vi "Sequencer Main - Copy.vi"() -> ()   [LabVIEW 2018] (continued)
                                # "Step TEST Result"
                                }
                                }
                                n2596 = global read "Global Variable.vi" "Array Errors"() -> (w5395:errorcluster[])
                                n2597 = Replace Array Subset(array=w5395, new element=w5392, index=3) -> (w5394:errorcluster[])
                                n2598 = global write "Global Variable.vi" "Array Errors"(w5394) -> ()
                                }
                              }
                            }
                            frame "capmem_get" {
                              # "Parameters"
                              # "Cmd"
                              n2599 = To Word Integer(number=w5406) -> (16bit integer=w5405:i16)
                              n2600 = To Word Integer(number=w5407) -> (16bit integer=w5404:i16)
                              n2601 = flat-sequence {
                                tunnel: [w5416] -> w5410
                                tunnel: [w5414] -> w5409
                                tunnel: [w5415] -> w5408
                                tunnel: w5410 -> [w5429]
                                tunnel: w5409 -> [w5428]
                                tunnel: w5408 -> [w5423]
                                tunnel: w5404 -> [w5427]
                                tunnel: w5405 -> [w5426]
                                tunnel: [w5425] -> w5403
                                tunnel: [w5424] -> w5402
                                tunnel: [w5422] -> w5399
                                tunnel: [w5421] -> w5398
                                frame #0 {
                                n2602 = global read "Global Variable.vi" "COM Port FTDI RS232"() -> (w5417:refnum<visa-resource-name>)
                                n2603 = call "ADB-Serial_WrRd.vi"("Timeout(Sec)"=1.0, "PassString"="Chuck(3)", "Command"="capmem", "ComPort"=w5417) -> ("error out"=w5415:errorcluster, "PASS"=w5416:bool, "received"=w5414:string)  [unwired: 5 in]
                                }
                                frame #1 {
                                n2604 = case shown="False" w5429 {
                                tunnel: w5428 -> [w5430 w5434]
                                tunnel: w5427 -> [_ w5439]
                                tunnel: w5426 -> [_ w5438]
                                tunnel: [FALSE w5437] -> w5425
                                tunnel: [w5432 w5436] -> w5424
                                tunnel: w5423 -> [w5432 w5436]
                                tunnel: [-1 w5435] -> w5422
                                tunnel: [w5430 w5434] -> w5421
                                frame False {
                                }
                                frame True {
                                n2605 = invoke on="Serial CMD Mon" class="Str" method="Append String"("string"=w5434) -> ()  [unwired: 3 in, 4 out]
                                n2606 = Match Pattern(string=w5434, regular expression="voltage") -> (after substring=w5443:string)  [unwired: 1 in, 3 out]
                                n2607 = Scan From String(format string="%d", input string=w5443, initial scan location=u32 0) -> (output 1=w5435:i32)  [unwired: 2 in, 3 out]
                                n2608 = In Range and Coerce(upper limit=w5439, x=w5435, lower limit=w5438) -> (In Range?=w5437:bool)  [unwired: 1 out]
                                }
                                }
                                }
                              }
                              n2609 = global read "Global Variable.vi" "Array Errors"() -> (w5411:errorcluster[])
                              n2610 = Replace Array Subset(array=w5411, new element=w5402, index=3) -> (w5412:errorcluster[])
                              n2611 = global write "Global Variable.vi" "Array Errors"(w5412) -> ()
                              n2612 = case shown="True" w5403 {
                                tunnel: [enum16{"Idle", "PASS", "FALSE"}."FALSE" ("Step Test Result") enum16{"Idle", "PASS", "FALSE"}."PASS" ("Step Test Result")] -> w5401
                                frame False {
                                # "Step TEST Result"
                                }
                                frame True {
                                # "Step TEST Result"
                                }
                              }
                              n2613 = Number To Decimal String(number=w5399) -> (decimal integer string=w5400:string)  [unwired: 1 in]
                            }
                            frame "setPowerRes" {
                              # "Param"
                              # "Cmd"
                              n2614 = flat-sequence {
                                tunnel: [w5457] -> w5452
                                tunnel: [w5456] -> w5451
                                tunnel: [w5455] -> w5450
                                tunnel: w5449 -> [w5454]
                                tunnel: w5452 -> [w5474]
                                tunnel: w5451 -> [w5475]
                                tunnel: [w5471] -> w5448
                                tunnel: w5450 -> [w5469]
                                tunnel: [w5470] -> w5447
                                tunnel: [w5469] -> w5446
                                frame #0 {
                                n2615 = for {
                                N: 1 -> [_]
                                tunnel: [w5459] -> w5457
                                tunnel: [w5468] -> w5456
                                shift-right: [w5458] -> w5455
                                shift-left: w5454 -> [w5463]
                                stop <- w5459 stop-if-true
                                n2616 = call <vilib>:"Space Constant.vi"() -> ("String"=w5462:string)
                                n2617 = global read "Global Variable.vi" "COM Port FTDI RS232"() -> (w5467:refnum<visa-resource-name>)
                                n2618 = Concatenate Strings("setPowerRes", w5462, w5463) -> (w5461:string)
                                n2619 = call "ADB-Serial_WrRd.vi"("Timeout(Sec)"=2.0, "PassString"="Set power resistor", "Command"=w5461, "ComPort"=w5467) -> ("error out"=w5468:errorcluster, "PASS"=w5459:bool, "received"=w5458:string)  [unwired: 5 in]
                                n2620 = invoke on="Serial CMD Mon" class="Str" method="Append String"("string"=w5458) -> ()  [unwired: 3 in, 4 out]
                                n2621 = Wait (ms)(milliseconds to wait=u32 500) -> ()  [unwired: 1 out]
                                }
                                }
                                frame #1 {
                                n2622 = global read "Global Variable.vi" "Array Errors"() -> (w5478:errorcluster[])
                                n2623 = call <userlib>:"Multi-line String to Array__ogtk.vi"("string"=w5469) -> ("lines"=w5473:string[])
                                n2624 = case shown="False" w5474 {
                                tunnel: [enum16{"Idle", "PASS", "FALSE"}."FALSE" ("Step Test Result") enum16{"Idle", "PASS", "FALSE"}."PASS" ("Step Test Result")] -> w5471
                                frame False {
                                # "Step TEST Result"
                                }
                                frame True {
                                # "Step TEST Result"
                                }
                                }
                                n2625 = Replace Array Subset(array=w5478, new element=w5475, index=3) -> (w5477:errorcluster[])
                                n2626 = Index Array(array=w5473, index=2 ("line index")) -> (element=w5470:string)
                                n2627 = global write "Global Variable.vi" "Array Errors"(w5477) -> ()
                                }
                              }
                            }
                            frame "calibADCoffset" {
                              # "Param"
                              # "Cmd"
                              n2628 = flat-sequence {
                                tunnel: [w5489] -> w5485
                                tunnel: [w5488] -> w5484
                                tunnel: [w5486] -> w5483
                                tunnel: w5485 -> [w5501]
                                tunnel: w5484 -> [w5502]
                                tunnel: [w5503] -> w5482
                                tunnel: w5483 -> [w5499]
                                tunnel: [w5499] -> w5481
                                frame #0 {
                                n2629 = for {
                                N: 1 -> [_]
                                tunnel: [w5493] -> w5489
                                tunnel: [w5498] -> w5488
                                tunnel: [w5490] -> w5486
                                stop <- w5493 stop-if-true
                                n2630 = global read "Global Variable.vi" "COM Port FTDI RS232"() -> (w5497:refnum<visa-resource-name>)
                                n2631 = global write "Global Variable.vi" "ADC Offset"(0 ("ADC Offset")) -> ()
                                n2632 = call "ADB-Serial_WrRd.vi"("Timeout(Sec)"=2.0, "PassString"="Chuck(3)", "Command"="calibADCoffset", "ComPort"=w5497) -> ("error out"=w5498:errorcluster, "PASS"=w5493:bool, "received"=w5490:string)  [unwired: 5 in]
                                n2633 = invoke on="Serial CMD Mon" class="Str" method="Append String"("string"=w5490) -> ()  [unwired: 3 in, 4 out]
                                n2634 = Wait (ms)(milliseconds to wait=u32 200) -> ()  [unwired: 1 out]
                                }
                                }
                                frame #1 {
                                n2635 = case shown="True" w5501 {
                                tunnel: w5499 -> [_ w5513]
                                tunnel: [FALSE w5508] -> w5500
                                frame False {
                                }
                                frame True {
                                n2636 = Match Pattern(string=w5513, regular expression="New ADC offset:") -> (after substring=w5511:string)  [unwired: 1 in, 3 out]
                                n2637 = Scan From String(format string="%d", input string=w5511) -> (output 1=w5509:i32)  [unwired: 3 in, 3 out]
                                n2638 = global write "Global Variable.vi" "ADC Offset"(w5509) -> ()
                                n2639 = Greater Than 0?(x=w5509) -> (x > 0?=w5508:bool)
                                }
                                }
                                n2640 = global read "Global Variable.vi" "Array Errors"() -> (w5506:errorcluster[])
                                n2641 = Replace Array Subset(array=w5506, new element=w5502, index=3) -> (w5505:errorcluster[])
                                n2642 = case shown="False" w5500 {
                                tunnel: [enum16{"Idle", "PASS", "FALSE"}."FALSE" ("Step Test Result") enum16{"Idle", "PASS", "FALSE"}."PASS" ("Step Test Result")] -> w5503
                                frame False {
                                # "Step TEST Result"
                                }
                                frame True {
                                # "Step TEST Result"
                                }
                                }
                                n2643 = global write "Global Variable.vi" "Array Errors"(w5505) -> ()
                                }
                              }
                            }
                            frame "calibCCRsave" {
                              # "Param"
                              # "Cmd"
                              n2644 = flat-sequence {
                                tunnel: [w5525] -> w5520
                                tunnel: [w5524] -> w5519
                                tunnel: w5518 -> [w5522]
                                tunnel: [w5521] -> w5516
                                tunnel: w5520 -> [w5539]
                                tunnel: w5519 -> [w5540]
                                tunnel: [w5537] -> w5517
                                frame #0 {
                                n2645 = for {
                                N: 1 -> [_]
                                tunnel: [w5531] -> w5525
                                tunnel: [w5536] -> w5524
                                tunnel: w5522 -> [w5528]
                                tunnel: [w5527] -> w5521
                                stop <- w5531 stop-if-true
                                (unwired) ""
                                n2646 = global read "Global Variable.vi" "COM Port FTDI RS232"() -> (w5535:refnum<visa-resource-name>)
                                n2647 = call <vilib>:"Space Constant.vi"() -> ("String"=w5526:string)
                                n2648 = Concatenate Strings("calibCCRsave", w5526, w5528) -> (w5529:string)
                                n2649 = call "ADB-Serial_WrRd.vi"("Timeout(Sec)"=2.0, "PassString"="Chuck(3)", "Command"=w5529, "ComPort"=w5535) -> ("error out"=w5536:errorcluster, "PASS"=w5531:bool, "received"=w5527:string)  [unwired: 5 in]
                                n2650 = invoke on="Serial CMD Mon" class="Str" method="Append String"("string"=w5527) -> ()  [unwired: 3 in, 4 out]
                                n2651 = Wait (ms)(milliseconds to wait=u32 200) -> ()  [unwired: 1 out]
                                }
                                }
                                frame #1 {
                                n2652 = global read "Global Variable.vi" "Array Errors"() -> (w5543:errorcluster[])
                                n2653 = case shown="True" w5539 {
                                tunnel: [FALSE w5545] -> w5538
                                frame False {
                                }
                                frame True {
                                n2654 = global read "Global Variable.vi" "ADC Offset"() -> (w5546:i32)
                                n2655 = Greater Than 0?(x=w5546) -> (x > 0?=w5545:bool)
                                }
                                }
                                n2656 = Replace Array Subset(array=w5543, new element=w5540, index=3) -> (w5542:errorcluster[])
                                n2657 = global write "Global Variable.vi" "Array Errors"(w5542) -> ()
                                n2658 = case shown="False" w5538 {
                                tunnel: [enum16{"Idle", "PASS", "FALSE"}."FALSE" ("Step Test Result") enum16{"Idle", "PASS", "FALSE"}."PASS" ("Step Test Result")] -> w5537
                                frame False {
                                # "Step TEST Result"
                                }
                                frame True {
                                # "Step TEST Result"
                                }
                                }
                                }
                              }
                            }
                            frame "start_ble" {
                              # "Param"
                              # "Cmd"
                              n2659 = flat-sequence {
                                tunnel: [w5558] -> w5554
                                tunnel: [w5557] -> w5553
                                tunnel: [w5555] -> w5551
                                tunnel: [w5555] -> w5549
                                tunnel: w5554 -> [w5571]
                                tunnel: w5553 -> [w5572]
                                tunnel: [w5573] -> w5552
                                tunnel: w5551 -> [w5570]
                                tunnel: [w5568] -> w5550
                                frame #0 {
                                n2660 = for {
                                N: 1 -> [_]
                                tunnel: [w5561] -> w5558
                                tunnel: [w5566] -> w5557
                                tunnel: [w5559] -> w5555
                                stop <- w5561 stop-if-true
                                n2661 = global read "Global Variable.vi" "COM Port FTDI RS232"() -> (w5565:refnum<visa-resource-name>)
                                n2662 = call "ADB-Serial_WrRd.vi"("Timeout(Sec)"=7.0, "PassString"="Chuck(3)", "Command"="start_ble", "ComPort"=w5565) -> ("error out"=w5566:errorcluster, "PASS"=w5561:bool, "received"=w5559:string)  [unwired: 5 in]
                                n2663 = invoke on="Serial CMD Mon" class="Str" method="Append String"("string"=w5559) -> ()  [unwired: 3 in, 4 out]
                                n2664 = Wait (ms)(milliseconds to wait=u32 200) -> ()  [unwired: 1 out]
                                }
                                }
                                frame #1 {
                                n2665 = global read "Global Variable.vi" "Array Errors"() -> (w5576:errorcluster[])
                                n2666 = call <userlib>:"Multi-line String to Array__ogtk.vi"("string"=w5570) -> ("lines"=w5569:string[])
                                n2667 = Index Array(array=w5569, index=4) -> (element=w5568:string)
                                n2668 = Replace Array Subset(array=w5576, new element=w5572, index=3) -> (w5575:errorcluster[])
                                n2669 = global write "Global Variable.vi" "Array Errors"(w5575) -> ()
                                n2670 = case shown="False" w5571 {
                                tunnel: [enum16{"Idle", "PASS", "FALSE"}."FALSE" ("Step Test Result") enum16{"Idle", "PASS", "FALSE"}."PASS" ("Step Test Result")] -> w5573
                                frame False {
                                # "Step TEST Result"
                                }
                                frame True {
                                # "Step TEST Result"
                                }
                                }
                                }
                              }
                            }
                            frame "setopvg" {
                              # "Param"
                              # "Cmd"
                              n2671 = flat-sequence {
                                tunnel: [w5589] -> w5584
                                tunnel: [w5588] -> w5583
                                tunnel: [w5586] -> w5581
                                tunnel: w5580 -> [w5585]
                                tunnel: w5584 -> [w5603]
                                tunnel: w5583 -> [w5604]
                                tunnel: [w5605] -> w5582
                                tunnel: w5581 -> [w5602]
                                tunnel: [w5602] -> w5579
                                frame #0 {
                                n2672 = for {
                                N: 1 -> [_]
                                tunnel: [w5596] -> w5589
                                tunnel: [w5601] -> w5588
                                tunnel: [w5591] -> w5586
                                tunnel: w5585 -> [w5593]
                                stop <- w5596 stop-if-true
                                n2673 = global read "Global Variable.vi" "COM Port FTDI RS232"() -> (w5600:refnum<visa-resource-name>)
                                n2674 = call <vilib>:"Space Constant.vi"() -> ("String"=w5594:string)
                                n2675 = Concatenate Strings("setopvg", w5594, w5593) -> (w5592:string)
                                n2676 = call "ADB-Serial_WrRd.vi"("Tx Deay"=u16 1, "Timeout(Sec)"=2.0, "PassString"="Chuck(3)", "Command"=w5592, "ComPort"=w5600) -> ("error out"=w5601:errorcluster, "PASS"=w5596:bool, "received"=w5591:string)  [unwired: 4 in]
                                n2677 = invoke on="Serial CMD Mon" class="Str" method="Append String"("string"=w5591) -> ()  [unwired: 3 in, 4 out]
                                n2678 = Wait (ms)(milliseconds to wait=u32 200) -> ()  [unwired: 1 out]
                                }
                                }
                                frame #1 {
                                n2679 = global read "Global Variable.vi" "Array Errors"() -> (w5608:errorcluster[])
                                n2680 = case shown="True" w5603 {
                                tunnel: [enum16{"Idle", "PASS", "FALSE"}."FALSE" ("Step Test Result") enum16{"Idle", "PASS", "FALSE"}."PASS" ("Step Test Result")] -> w5605
                                frame False {
                                # "Step TEST Result"
                                }
                                frame True {
                                # "Step TEST Result"
                                }
                                }
                                n2681 = Replace Array Subset(array=w5608, new element=w5604, index=3) -> (w5607:errorcluster[])
                                n2682 = global write "Global Variable.vi" "Array Errors"(w5607) -> ()
                                }
                              }
                            }
                            frame "reset" {
                              # "Param"
                              # "Cmd"
                              n2683 = flat-sequence {
                                tunnel: [w5619] -> w5615
                                tunnel: [w5618] -> w5614
                                tunnel: [w5616] -> w5611
                                tunnel: w5615 -> [w5629]
                                tunnel: w5614 -> [w5630]
                                tunnel: [w5631] -> w5613
                                tunnel: [w5628] -> w5612
                                tunnel: w5611 -> [w5628]
                                frame #0 {
                                n2684 = for {
                                N: 1 -> [_]
                                tunnel: [w5623] -> w5619
                                tunnel: [w5627] -> w5618
                                tunnel: [w5620] -> w5616
                                stop <- w5623 stop-if-true
                                n2685 = global read "Global Variable.vi" "COM Port FTDI RS232"() -> (w5626:refnum<visa-resource-name>)
                                n2686 = call "ADB-Serial_WrRd.vi"("Timeout(Sec)"=2.0, "PassString"="", "Command"="reset", "ComPort"=w5626) -> ("error out"=w5627:errorcluster, "PASS"=w5623:bool, "received"=w5620:string)  [unwired: 5 in]
                                n2687 = invoke on="Serial CMD Mon" class="Str" method="Append String"("string"=w5620) -> ()  [unwired: 3 in, 4 out]
                                n2688 = Wait (ms)(milliseconds to wait=u32 500) -> ()  [unwired: 1 out]
                                }
                                }
                                frame #1 {
                                n2689 = global read "Global Variable.vi" "Array Errors"() -> (w5634:errorcluster[])
                                n2690 = case shown="True" w5629 {
                                tunnel: [enum16{"Idle", "PASS", "FALSE"}."FALSE" ("Step Test Result") enum16{"Idle", "PASS", "FALSE"}."PASS" ("Step Test Result")] -> w5631
                                frame False {
                                # "Step TEST Result"
                                }
                                frame True {
                                # "Step TEST Result"
                                }
                                }
                                n2691 = Replace Array Subset(array=w5634, new element=w5630, index=3) -> (w5633:errorcluster[])
                                n2692 = global write "Global Variable.vi" "Array Errors"(w5633) -> ()
                                }
                              }
                            }
                          }
                          n2693 = local read "Debugging"() -> (w4491:bool)
                          n2694 = in-place {
                            in-place-border: w4492 -> [w4535]
                            in-place-border: [w4534] -> w4488
                            in-place-border: [w4533] -> w4489
                            # "GoTo Test-nmb"
                            # "ReTest Cyckles"
                            n2695 = Index Array(array=w4535, index #1=0, index #2=1, index #3=2) -> (element #2=w4539:string, element #3=w4540:string)  [unwired: 1 out]
                            n2696 = Decimal String To Number(string=w4539) -> (number=w4534:i32)  [unwired: 2 in, 1 out]
                            n2697 = Decimal String To Number(string=w4540) -> (number=w4533:i32)  [unwired: 2 in, 1 out]
                          }
                          n2698 = case shown="False" w4491 {
                            tunnel: w4490 -> [w4520 _]
                            tunnel: w4488 -> [w4518 _]
                            tunnel: w4489 -> [w4517 _]
                            frame False {
                              # "No Debug Mode"
                              n2699 = in-place {
                                in-place-border: [w4522] -> w4519
                                n2700 = global read "Global Variable.vi" "Retest Cnt"() -> (w4523:i16)
                                n2701 = Equal?(x=w4523, y=i16 0) -> (x = y?=w4522:bool)
                              }
                              n2702 = case shown="True" w4520 {
                                tunnel: w4519 -> [_ w4527]
                                tunnel: w4518 -> [_ w4525]
                                tunnel: w4517 -> [_ w4524]
                                frame False {
                                }
                                frame True {
                                # "String \"false\" Present"
                                n2703 = global write "Global Variable.vi" "Retest Step Nmb"(w4525) -> ()
                                n2704 = global write "Global Variable.vi" "Retest Nmb"(w4524) -> ()
                                n2705 = case shown="False" w4527 {
                                tunnel: w4524 -> [_ w4532]
                                frame False {
                                n2706 = global read "Global Variable.vi" "Retest Cnt"() -> (w4530:i16)
                                n2707 = Decrement(x=w4530) -> (x-1=w4529:i16)
                                n2708 = global write "Global Variable.vi" "Retest Cnt"(w4529) -> ()
                                n2709 = Wait (ms)(milliseconds to wait=u32 1000) -> ()  [unwired: 1 out]
                                }
                                frame True {
                                # "if(Retest-OFF & Cnt=0)"
                                n2710 = Decrement(x=w4532) -> (x-1=w4531:i32)
                                n2711 = global write "Global Variable.vi" "Retest Cnt"(w4531) -> ()
                                }
                                }
                                n2712 = global write "Global Variable.vi" "Retest ON"(TRUE ("Retest ON")) -> ()
                                }
                              }
                            }
                            frame True {
                            }
                          }
                          n2713 = in-place {
                            in-place-border: w4482 -> [w4514]
                            in-place-border: w4483 -> [w4513]
                            in-place-border: w4484 -> [w4512]
                            n2714 = call "Log Add Msg.vi"("Result"=w4512, "Communication"=w4513, "Description"=w4514) -> ("Out Msg"=w4515:string)
                            n2715 = property on="LogMsg" class="Str"("Text.Scroll Position"=inf) -> ()  [unwired: 2 in, 2 out]
                            n2716 = invoke on="LogMsg" class="Str" method="Append String"("string"=w4515) -> ()  [unwired: 3 in, 4 out]
                          }
                        }
                        frame 70 {
                          w5644 = "\r\n"
                          # "Step TEST Result"
                          # "FLASH Case"
                          # "FLASH Case"
                          n2717 = Unbundle By Name(w5649) -> ("Step Description"=w5639:string, "Parameters"=w5645:string)  [unwired: 1 out]
                          n2718 = Concatenate Strings("FLASH ADB Board", w5644, w5645, w5644) -> (w5643:string)
                          n2719 = invoke on="Msg Str" class="Str" method="Append String"("string"=w5643) -> (error out=w5642:errorcluster)  [unwired: 3 in, 3 out]
                          n2720 = property on="Tab Control Msg" class="TabCtl (strict)"("Value"=T21."Msg" ("Tab Control Msg")) -> (error out=w5647:errorcluster)  [unwired: 2 in, 1 out]
                          n2721 = in-place {
                            in-place-border: w5647 -> [_]
                            in-place-border: w5645 -> [w5665]
                            in-place-border: w5642 -> [_]
                            in-place-border: [w5660] -> w5641
                            in-place-border: [w5659] -> w5638
                            n2722 = call "Flash_ADB.vi"("Flash Bat File"=w5665) -> ("error out"=w5661:errorcluster, "standard output"=w5659:string, "Result"=w5660:bool)  [unwired: 7 in, 1 out]
                            n2723 = global read "Global Variable.vi" "Array Errors"() -> (w5663:errorcluster[])
                            n2724 = invoke on="Msg Str" class="Str" method="Append String"("string"=w5659) -> ()  [unwired: 3 in, 4 out]
                            n2725 = Replace Array Subset(array=w5663, new element=w5661, index=10) -> (w5664:errorcluster[])
                            n2726 = global write "Global Variable.vi" "Array Errors"(w5664) -> ()
                          }
                          n2727 = case shown="True" w5641 {
                            tunnel: [enum16{"Idle", "PASS", "FALSE"}."FALSE" ("Step Test Result") enum16{"Idle", "PASS", "FALSE"}."PASS" ("Step Test Result")] -> w5640
                            tunnel: ["FLASH FALSE" "FLASH OK"] -> w5637
                            frame False {
                              # "Step TEST Result"
                            }
                            frame True {
                              # "Step TEST Result"
                            }
                          }
                          n2728 = in-place {
                            in-place-border: w5639 -> [w5652]
                            in-place-border: w5638 -> [w5651]
                            in-place-border: w5637 -> [w5650]
                            n2729 = call "Log Add Msg.vi"("Result"=w5650, "Communication"=w5651, "Description"=w5652) -> ("Out Msg"=w5653:string)
                            n2730 = property on="LogMsg" class="Str"("Text.Scroll Position"=inf) -> ()  [unwired: 2 in, 2 out]
                            n2731 = invoke on="LogMsg" class="Str" method="Append String"("string"=w5653) -> ()  [unwired: 3 in, 4 out]
                          }
                        }
                        frame 1000 {
                          # "Power Supply OFF, Reset DIO"
                          # "Step TEST Result"
                          # "RESET POWER SUPPLY & RESET GPIO"
                          n2732 = Unbundle By Name(w5674) -> ("Step Description"=w5673:string)
                          n2733 = Concatenate Strings(w5673, "  " ("string"), "<END OF SEQUENCER>" ("string")) -> (w5675:string)
                          n2734 = local write "Message"(w5675) -> ()
                          n2735 = property on="Tab Control Msg" class="TabCtl (strict)"("Value"=T21."Msg" ("Tab Control Msg")) -> (error out=w5668:errorcluster)  [unwired: 2 in, 1 out]
                          n2736 = flat-sequence {
                            tunnel: w5668 -> [_]
                            tunnel: w5667 -> [w5693]
                            tunnel: w5666 -> [w5692]
                            frame #0 {
                              w5678 = FALSE ("Enable Output")
                              w5676 = 0.1 ("Current")
                              w5677 = 0.0 ("Voltage")
                              n2737 = global read "Global Variable.vi" "VISA Resource Name BK-9202"() -> (w5687:string)
                              n2738 = call "bk9201 Set.vi"("Enable Output"=w5678, "Current"=w5676, "Voltage"=w5677, "VISA resource name"=w5687) -> ("error out"=w5683:errorcluster)  [unwired: 7 in]
                              n2739 = local read "PowSupply - SET"() -> (w5680:T7)
                              n2740 = local read "Switch Relay Modules"() -> (w5682:T5)
                              n2741 = Bundle By Name(cluster=w5682, "Main Power Supplay ON/OFF"=w5678) -> (w5681:T5)
                              n2742 = global read "Global Variable.vi" "Array Errors"() -> (w5685:errorcluster[])
                              n2743 = Bundle By Name(cluster=w5680, "ON/OFF"=w5678, "Volt (V)"=w5677, "Current Limit (A)"=w5676) -> (w5679:T7)
                              n2744 = global write "Global Variable.vi" "PowSupply ON/OFF"(w5678) -> ()
                              n2745 = Replace Array Subset(array=w5685, new element=w5683, index=2) -> (w5686:errorcluster[])
                              n2746 = local write "Switch Relay Modules"(w5681) -> ()
                              n2747 = local write "PowSupply - SET"(w5679) -> ()
                              n2748 = global write "Global Variable.vi" "Array Errors"(w5686) -> ()
                            }
                            frame #1 {
                              n2749 = call <vilib>:"Acquire Semaphore.vi"("error in (no error)"=w5693, "semaphore"=w5692) -> ("error out"=w5691:errorcluster, "semaphore out"=w5689:T13)  [unwired: 3 in, 1 out]
                              n2750 = case shown="No Error" w5691 {
                                selector: w5691 -> [w5695 w5714]
                                tunnel: [w5695 w5714] -> w5688
                                tunnel: [w5694 w5713] -> w5690
                                tunnel: w5689 -> [w5694 w5713]
                                frame No Error {
                                n2751 = disable-structure shown="Disabled" {
                                frame Disabled {
                                n2752 = local read "Switch Relay Modules"() -> (w5703:T5)
                                n2753 = Number To Boolean Array(number=u16 0) -> (Boolean array=w5705:bool[])
                                n2754 = Bundle By Name(cluster=w5703, "SW 0"=w5705, "SW 1"=w5705, "SW 2"=w5705, "SW 3"=w5705, "SW 4"=w5705, "SW 5"=w5705, "SW 6"=w5705) -> (w5704:T5)
                                n2755 = local write "Switch Relay Modules"(w5704) -> ()
                                }
                                frame Enabled {
                                }
                                }
                                n2756 = global read "Global Variable.vi" "FTDI SPI Handle"() -> (w5698:u32)
                                n2757 = for {
                                N: 7 -> [_]
                                tunnel: w5698 -> [w5711]
                                tunnel: [w5712] -> w5701
                                i -> [w5706]
                                w5708 = u8 0  # nCS
                                w5707 = u16 0  # Channel Decimal
                                w5709 = FALSE  # Use Extra
                                n2758 = call "FTDI SPI GPIO Set.vi"("nCS"=w5708, "Mode"=T23."Set Decimal", "Use Extra"=w5709, "Channel Decimal"=w5707, "Addr"=w5706, "Handler In"=w5711) -> ("error out"=w5712:errorcluster)  [unwired: 2 in, 3 out]
                                }
                                n2759 = global read "Global Variable.vi" "Array Errors"() -> (w5699:errorcluster[])
                                n2760 = Replace Array Subset(array=w5699, new element=w5701, index=10) -> (w5700:errorcluster[])
                                n2761 = global write "Global Variable.vi" "Array Errors"(w5700) -> ()
                                }
                                frame Error {
                                }
                              }
                              n2762 = call <vilib>:"Release Semaphore.vi"("error in (no error)"=w5688, "semaphore"=w5690) -> ()  [unwired: 4 in, 2 out]
                            }
                            frame #2 {
                              w5715 = "!END OF TEST\nReset ALL"
                              n2763 = local write "Message"(w5715) -> ()
                              n2764 = property on="Msg Str" class="Str"("Value"=w5715) -> ()  [unwired: 2 in, 2 out]
                            }
                          }
                        }
                      }
                    }
                  }
                }
                frame #1 {
                  # "Step Result Msg"
                  # "Report"
                  # "Step TEST Result"
                  # "Run/Skip"
                  # "Step Type"
                  # "PASS/FALSE"
                  n2765 = Unbundle By Name(w5730) -> ("Run/Skip"=w5726:bool, "Step Type"=w5729:u16, "Report"=w5718:bool)
                  n2766 = flat-sequence {
                    tunnel: w5723 -> [w5735]
                    tunnel: w5716 -> [w5736]
                    tunnel: [w5738] -> w5728
                    tunnel: [w5737] -> w5727
                    tunnel: w5725 -> [w5733]
                    tunnel: [w5734] -> w5721
                    tunnel: w5728 -> [w5780]
                    tunnel: w5727 -> [w5781]
                    tunnel: w5716 -> [w5786]
                    tunnel: w5726 -> [w5782]
                    tunnel: w5724 -> [w5785]
                    tunnel: [w5784] -> w5717
                    tunnel: [w5783] -> w5722
                    tunnel: w5721 -> [w5783]
                    tunnel: w5716 -> [w5818]
                    tunnel: w5723 -> [w5817]
                    tunnel: w5722 -> [w5813]
                    tunnel: [w5812] -> w5719
                    tunnel: [w5847] -> w5720
                    tunnel: w5719 -> [w5847]
                    frame #0 {
                      # "BREACK ON FIRST Err"
                      n2767 = flat-sequence {
                        tunnel: w5733 -> [w5740]
                        tunnel: w5735 -> [w5741]
                        tunnel: w5736 -> [w5739]
                        tunnel: [w5741] -> w5732
                        tunnel: [w5740] -> w5731
                        tunnel: [w5752] -> w5738
                        tunnel: [w5751] -> w5737
                        tunnel: [w5749] -> w5734
                        tunnel: w5732 -> [w5750]
                        tunnel: w5731 -> [w5748]
                        frame #0 {
                          n2768 = case shown="\"FALSE\"" w5739 {
                            frame "Idle", Default {
                            }
                            frame "FALSE" {
                              n2769 = in-place {
                                in-place-border: [w5743] -> w5742
                                n2770 = global read "Global Variable.vi" "Retest Cnt"() -> (w5744:i16)
                                n2771 = Equal?(x=w5744, y=i16 0) -> (x = y?=w5743:bool)
                              }
                              n2772 = case shown="True" w5742 {
                                frame False {
                                }
                                frame True {
                                n2773 = global read "Global Variable.vi" "Gen Err Cnt"() -> (w5747:u16)
                                n2774 = Increment(x=w5747) -> (x+1=w5746:u16)
                                n2775 = global write "Global Variable.vi" "Gen Err Cnt"(w5746) -> ()
                                }
                              }
                            }
                          }
                        }
                        frame #1 {
                          # "GoTo  the last Sekuencer STEP (test Id=1000)"
                          n2776 = in-place {
                            in-place-border: [w5764] -> w5749
                            in-place-border: [w5762] -> w5752
                            in-place-border: [w5761] -> w5751
                            in-place-border: w5750 -> [w5760]
                            in-place-border: w5748 -> [w5759]
                            # "And"
                            # "Break On 3xFirst Err"
                            n2777 = global read "Global Variable.vi" "Gen Err Cnt"() -> (w5758:u16)
                            n2778 = Greater Or Equal?(x=w5758, y=u16 3) -> (x >= y?=w5754:bool)
                            n2779 = And(x=w5754, y="Break On First Err") -> (x .and. y?=w5755:bool)
                            n2780 = case shown="True" w5755 {
                              tunnel: [FALSE TRUE] -> w5756
                              frame False {
                              }
                              frame True {
                                n2781 = global write "Global Variable.vi" "Test Gen Status"(FALSE ("Test Gen Status")) -> ()
                              }
                            }
                            n2782 = And(x=w5756, y="Break On First Err") -> (x .and. y?=w5763:bool)
                            n2783 = case shown="True" w5763 {
                              tunnel: w5760 -> [_ w5778]
                              tunnel: w5759 -> [w5770 w5779]
                              tunnel: [w5770 w5775] -> w5764
                              tunnel: [FALSE TRUE] -> w5762
                              tunnel: [0 w5771] -> w5761
                              frame False {
                              }
                              frame True {
                                n2784 = global read "Sequencer Array.vi" "SEQUENCER Array"() -> (w5777:T16[])
                                n2785 = Flush Queue(queue=w5778, error in (no error)=w5779) -> (queue out=w5776:refnum<queue>, error out=w5774:errorcluster)  [unwired: 1 out]
                                n2786 = Array Size(array=w5777) -> (size(s)=w5773:i32)
                                n2787 = Decrement(x=w5773) -> (x-1=w5771:i32)
                                n2788 = property on="Test Sequencer" class="MCListbox (strict)"("Value"=w5771) -> ()  [unwired: 2 in, 2 out]
                                n2789 = Enqueue Element(queue=w5776, element=w5771, error in (no error)=w5774) -> (error out=w5775:errorcluster)  [unwired: 1 in, 2 out]
                              }
                            }
                          }
                        }
                      }
                    }
                    frame #1 {
                      # "Step TEST Result"
                      # "Run/Skip & Retest-ON"
                      # "Fill-Up (PASS/FALSE)Test Sequenser Table"
                      n2790 = case shown="True" w5780 {
                        tunnel: w5781 -> [_ w5789]
                        frame False {
                        }
                        frame True {
                          # "Break on first Err jump"
                          n2791 = Add(x=w5789, y=-5) -> (x+y=w5788:i32)
                          n2792 = Bundle By Name(cluster=T14 {"Row"=0, "Column"=0} ("Top Left Visible Cell"), "Row"=w5788, "Column"=u32 0) -> (w5792:T14)
                          n2793 = property on="Test Sequencer" class="MCListbox (strict)"("TopLeft"=w5792) -> ()  [unwired: 2 in, 2 out]
                        }
                      }
                      n2794 = case shown="True" w5782 {
                        tunnel: w5786 -> [_ w5801]
                        tunnel: [u32 16448250 w5797] -> w5784
                        tunnel: w5785 -> [_ w5794]
                        frame False {
                        }
                        frame True {
                          w5802 = 5 ("disabled index (col)")
                          # "Step Result Msg"
                          # "A-1"
                          n2795 = case shown="\"FALSE\"" w5801 {
                            tunnel: [u32 16448250 u32 46115 u32 16711680] -> w5797
                            tunnel: ["Idle" "PASS" "FALSE"] -> w5800
                            frame "Idle", Default {
                            }
                            frame "PASS" {
                            }
                            frame "FALSE" {
                            }
                          }
                          n2796 = global read "Global Variable.vi" "Current Step Nmb"() -> (w5796:u32)
                          n2797 = property on="Test Squencer Edit" class="MCListbox (strict)"() -> ("ItemNames"=w5798:string[][])  [unwired: 2 in, 2 out]
                          n2798 = Bundle By Name(cluster=T15 {"Row"=0, "Column"=0} ("Active Cell:Active Cell"), "Row"=w5796, "Column"=w5802) -> (w5803:T15)
                          n2799 = Replace Array Subset(array=w5798, new element #1=w5800, index (row) #1=w5796, index (col) #1=w5802, new element #2=w5794, index (row) #2=w5796, index (col) #2=3 ("disabled index (col)")) -> (w5799:string[][])
                          n2800 = property on="Test Squencer Edit" class="MCListbox (strict)"("ItemNames"=w5799, "ActiveCell"=w5803, "CellFontColor"=w5797) -> ()  [unwired: 2 in, 2 out]
                        }
                      }
                    }
                    frame #2 {
                      # "Step TEST Result"
                      n2801 = global read "Global Variable.vi" "Retest Cnt"() -> (w5811:i16)
                      n2802 = global read "Global Variable.vi" "Retest ON"() -> (w5815:bool)
                      n2803 = Greater Than 0?(x=w5811) -> (x > 0?=w5814:bool)
                      n2804 = And(x=w5815, y=w5814) -> (x .and. y?=w5816:bool)
                      n2805 = case shown="True" w5816 {
                        tunnel: w5818 -> [_ w5823]
                        tunnel: w5817 -> [_ w5822]
                        tunnel: w5813 -> [w5819 w5821]
                        tunnel: [w5819 w5820] -> w5812
                        frame False {
                        }
                        frame True {
                          n2806 = case shown="\"FALSE\"" w5823 {
                            tunnel: [w5824 w5827 w5845] -> w5820
                            tunnel: w5822 -> [_ w5826 _]
                            tunnel: w5821 -> [w5824 w5825 w5845]
                            frame "Idle", Default {
                            }
                            frame "FALSE" {
                              n2807 = in-place {
                                in-place-border: w5826 -> [w5835]
                                in-place-border: w5825 -> [w5834]
                                in-place-border: [w5829] -> w5827
                                # "RETEST"
                                n2808 = global read "Global Variable.vi" "Retest Step Nmb"() -> (w5828:u32)
                                n2809 = global read "Global Variable.vi" "Steps Nmb"() -> (w5831:u32)
                                n2810 = disable-structure shown="Disabled" {
                                disable-tunnel: w5828 -> [w5836 _]
                                frame Disabled {
                                n2811 = Bundle By Name(cluster=T14 {"Row"=0, "Column"=0} ("Top Left Visible Cell"), "Row"=w5836) -> (w5837:T14)
                                n2812 = property on="Test Sequencer" class="MCListbox (strict)"("TopLeft"=w5837) -> ()  [unwired: 2 in, 2 out]
                                }
                                frame Enabled {
                                }
                                }
                                n2813 = Flush Queue(queue=w5835, error in (no error)=w5834) -> (queue out=w5832:refnum<queue>, error out=w5833:errorcluster)  [unwired: 1 out]
                                n2814 = property on="Test Sequencer" class="MCListbox (strict)"("Value"=w5828) -> ()  [unwired: 2 in, 2 out]
                                n2815 = Subtract(x=w5831, y=w5828) -> (x-y=w5830:u32)
                                n2816 = for {
                                N: w5830 -> [_]
                                tunnel: w5833 -> [w5844]
                                tunnel: w5832 -> [w5843]
                                tunnel: w5828 -> [w5840]
                                tunnel: [w5839] -> w5829
                                i -> [w5842]
                                n2817 = Add(x=w5840, y=w5842) -> (x+y=w5841:u32)
                                n2818 = Enqueue Element(queue=w5843, element=w5841, error in (no error)=w5844) -> (error out=w5839:errorcluster)  [unwired: 1 in, 2 out]
                                }
                              }
                            }
                            frame "PASS" {
                              n2819 = global write "Global Variable.vi" "Retest Cnt"(i16 0 ("Retest Cnt")) -> ()
                            }
                          }
                        }
                      }
                    }
                    frame #3 {
                      n2820 = in-place {
                        n2821 = global read "Global Variable.vi" "Retest Nmb"() -> (w5848:i16)
                        n2822 = global read "Global Variable.vi" "Retest Cnt"() -> (w5850:i16)
                        n2823 = Subtract(x=w5848, y=w5850) -> (x-y=w5849:i16)
                        n2824 = Number To Decimal String(number=w5849) -> (decimal integer string=w5852:string)  [unwired: 1 in]
                        n2825 = Greater Than 0?(x=w5850) -> (x > 0?=w5853:bool)
                        "RETEST" <- w5853
                        n2826 = global write "Global Variable.vi" "Retest ON"(FALSE ("Retest Start")) -> ()
                        n2827 = case shown="False" w5853 {
                          tunnel: w5852 -> [w5854 w5855]
                          frame False {
                            n2828 = property on="RETEST" class="Bool (strict)"("BoolText.Text"=w5854) -> ()  [unwired: 2 in, 2 out]
                          }
                          frame True {
                            n2829 = property on="RETEST" class="Bool (strict)"("BoolText.Text"=w5855) -> ()  [unwired: 2 in, 2 out]
                          }
                        }
                      }
                    }
                  }
                }
                frame #2 {
                  # "Report"
                  # "Run / Skip"
                  # "A-1"
                  # "REPORT GENERATION"
                  n2830 = global read "Global Variable.vi" "Retest Cnt"() -> (w5860:i16)
                  n2831 = Equal To 0?(x=w5860) -> (x = 0?=w5858:bool)
                  n2832 = in-place {
                    in-place-border: w5862 -> [w5865]
                    # "Error Store"
                    n2833 = global read "Global Variable.vi" "Array Errors"() -> (w5867:errorcluster[])
                    n2834 = Replace Array Subset(array=w5867, new element=w5865, index=7) -> (w5868:errorcluster[])
                    n2835 = global write "Global Variable.vi" "Array Errors"(w5868) -> ()
                  }
                  n2836 = Compound Arithmetic op=AND(w5858, w5857, w5856) -> (w5859:bool)
                  n2837 = case shown="True" w5859 {
                    tunnel: w5864 -> [_ w5871]
                    tunnel: w5863 -> [_ w5870]
                    tunnel: w5861 -> [_ w5869]
                    frame False {
                    }
                    frame True {
                      n2838 = case shown="0" w5871 {
                        tunnel: w5870 -> [w5881 _ w5900]
                        tunnel: w5869 -> [w5877 _ _]
                        frame 100, Default {
                          # "All Steps (no Label)"
                          n2839 = case shown="\"FALSE\"" w5877 {
                            frame "Idle", Default {
                            }
                            frame "PASS" {
                            }
                            frame "FALSE" {
                              w5892 = u32 16746656
                              n2840 = Bundle(w5892, w5892) -> (w5893:cluster{u32, u32})  [unwired: 1 in]
                              n2841 = global write "Global Variable.vi" "Test Gen Status"(FALSE ("Test Gen Status")) -> ()
                              n2842 = Build Array(w5893) -> (w5894:cluster{u32, u32}[])
                              n2843 = property on="Gen Test Status" class="Bool (strict)"("Colors [4]"=w5894, "Value"=FALSE ("Gen Test Status")) -> ()  [unwired: 2 in, 2 out]
                            }
                          }
                          n2844 = global read "Global Variable.vi" "Current Step Nmb"() -> (w5888:u32)
                          n2845 = property on="Test Squencer Edit" class="MCListbox (strict)"() -> ("ItemNames"=w5889:string[][])  [unwired: 2 in, 2 out]
                          n2846 = global read "Global Variable.vi" "Report Step Nmb"() -> (w5879:u32)
                          n2847 = property on="Test Sequencer Run" class="MCListbox (strict)"() -> ("ItemNames"=w5887:string[][])  [unwired: 2 in, 2 out]
                          n2848 = Index Array(array=w5889, index (row)=w5888) -> (element=w5885:string[])  [unwired: 1 in]
                          n2849 = Increment(x=w5879) -> (x+1=w5878:u32)
                          n2850 = Number To Decimal String(number=w5879) -> (decimal integer string=w5876:string)  [unwired: 1 in]
                          n2851 = Replace Array Subset(array=w5885, new element=w5876, index=0) -> (w5875:string[])
                          n2852 = Array Subset(array=w5875, index=0, length=7) -> (w5872:string[])
                          n2853 = Bundle By Name(cluster=T15 {"Row"=0, "Column"=0} ("Active Cell:Active Cell"), "Row"=w5879, "Column"=5) -> (w5882:T15)
                          n2854 = Replace Array Subset(array=w5887, new element=w5872, index (row)=w5879) -> (w5886:string[][])  [unwired: 1 in]
                          n2855 = global write "Global Variable.vi" "Report Step Nmb"(w5878) -> ()
                          n2856 = property on="Test Sequencer Run" class="MCListbox (strict)"("ItemNames"=w5886, "ActiveCell"=w5882, "CellFontColor"=w5881, "Value"=w5879) -> ()  [unwired: 2 in, 2 out]
                        }
                        frame 1 {
                        }
                        frame 0 {
                          n2857 = global read "Global Variable.vi" "Current Step Nmb"() -> (w5911:u32)
                          n2858 = property on="Test Squencer Edit" class="MCListbox (strict)"() -> ("ItemNames"=w5912:string[][])  [unwired: 2 in, 2 out]
                          n2859 = global read "Global Variable.vi" "Report Step Nmb"() -> (w5902:u32)
                          n2860 = property on="Test Sequencer Run" class="MCListbox (strict)"() -> ("ItemNames"=w5910:string[][])  [unwired: 2 in, 2 out]
                          n2861 = Number To Decimal String(number=w5902) -> (decimal integer string=w5905:string)  [unwired: 1 in]
                          n2862 = for {
                            N: 7 -> [_]
                            tunnel: w5902 -> [w5915]
                            i -> [w5916]
                            n2863 = Bundle By Name(cluster=T15 {"Row"=0, "Column"=0} ("Active Cell:Active Cell"), "Row"=w5915, "Column"=w5916) -> (w5914:T15)
                            n2864 = property on="Test Sequencer Run" class="MCListbox (strict)"("ActiveCell"=w5914, "CellBG"=u32 16772930) -> ()  [unwired: 2 in, 2 out]
                          }
                          n2865 = Index Array(array=w5912, index (row)=w5911) -> (element=w5907:string[])  [unwired: 1 in]
                          n2866 = Increment(x=w5902) -> (x+1=w5908:u32)
                          n2867 = Replace Array Subset(array=w5907, new element=w5905, index=0) -> (w5897:string[])
                          n2868 = global write "Global Variable.vi" "Report Step Nmb"(w5908) -> ()
